vi "ShutdownFGV.vi"(8 "error in (no error)":errorcluster, 9 "Enum":enum16{"Set", "Get"}(ring), 11 "stop":bool) -> (0 "error in (no error) 2":errorcluster, 3 "Boolean":bool)   [LabVIEW 2020]
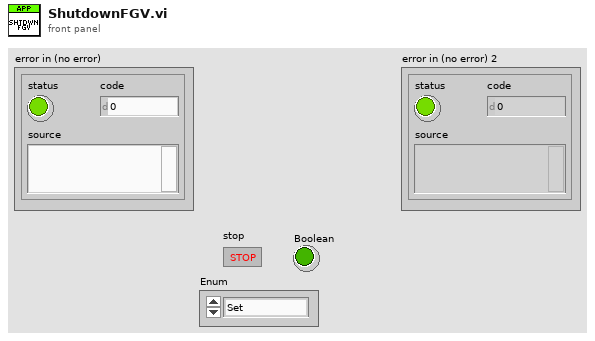
[diagram p1: front panel]
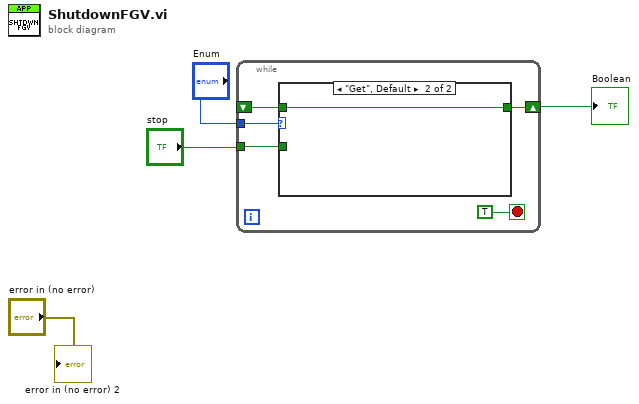
[diagram p0: block diagram]
diagram:
  n1 = while {
    shift-right: [w6] -> w3
    shift-left: _ -> [w5]
    tunnel: "stop" -> [w7]
    tunnel: "Enum" -> [w8]
    stop <- TRUE stop-if-true
    n2 = case shown="\"Get\", Default" w8 {
      tunnel: w7 -> [w10 _]
      tunnel: [w10 w11] -> w6
      tunnel: w5 -> [_ w11]
      frame "Set" {
      }
      frame "Get", Default {
      }
    }
  }
  "Boolean" <- w3
  "error in (no error) 2" <- "error in (no error)"
